vi "runup_main_data.vi"(6 "E RPM":dbl, 7 "running":bool, 9 "time_sec":u8, 10 "end_RPM":u16, 11 "start_RPM":u16) -> (1 "Numeric 3":dbl, 2 "Numeric":u8, 3 "Numeric 2":dbl, 4 "Boolean":bool)   [LabVIEW 2014]
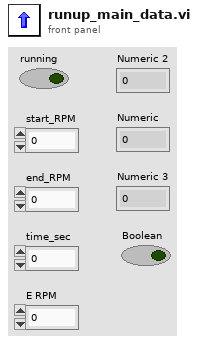
[diagram p1: front panel]
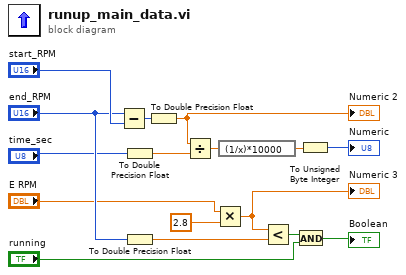
[diagram p0: block diagram]
diagram:
  n1 = Subtract(x="end_RPM", y="start_RPM") -> (x-y=w1:u16)
  n2 = To Double Precision Float(number="time_sec") -> (double precision float=w3:dbl)
  n3 = To Double Precision Float(number="end_RPM") -> (double precision float=w13:dbl)
  n4 = To Double Precision Float(number=w1) -> (double precision float=w8:dbl)
  "Numeric 2" <- w8
  n5 = Divide(x=w8, y=w3) -> (x/y=w9:dbl)
  n6 = Multiply(x="E RPM", y=2.8) -> (x*y=w7:dbl)
  "Numeric 3" <- w7
  n7 = expression code="(1/x)*10000"(w9) -> (w14:dbl)
  n8 = Less?(x=w7, y=w13) -> (x < y?=w4:bool)
  n9 = And(x=w4, y="running") -> (x .and. y?=→"Boolean":bool)
  n10 = To Unsigned Byte Integer(number=w14) -> (unsigned 8bit integer=→"Numeric":u8)
